vi "Close.vi"(8 "error in (no error)":errorcluster, 11 "PXI 4110 in":refnum<class "PXI 4110.lvclass">) -> (0 "error out":errorcluster, 3 "PXI 4110 out":refnum<class "PXI 4110.lvclass">)   [LabVIEW 2015, in "PXI 4110.lvclass"]
uses:
  PXI 4110.lvclass
  <userlib>/Common Components/Hardware/PSU/PSU.lvclass
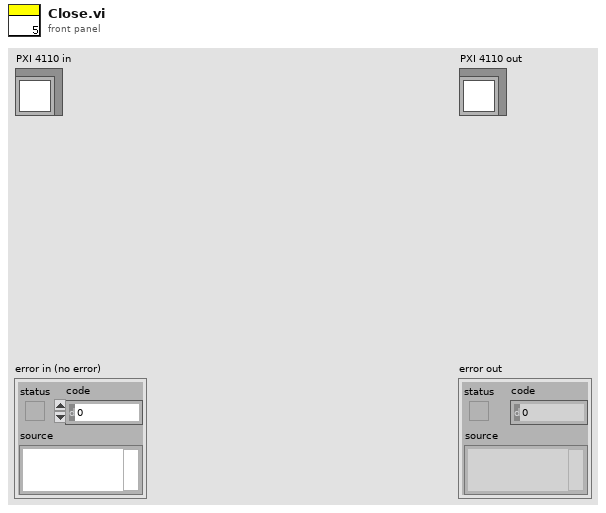
[diagram p1: front panel]
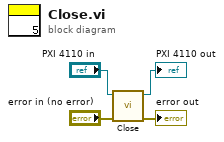
[diagram p0: block diagram]
diagram:
  n1 = call-parent "Close.vi"("error in (no error)"="error in (no error)", "PSU in"="PXI 4110 in") -> ("error out"=→"error out":errorcluster, "PSU out"=→"PXI 4110 out":refnum<class "PXI 4110.lvclass">)  [unwired: 8 in]
